vi "UpDownBinaryCounter12bitBreadmore.vi"() -> ()   [LabVIEW 2020]
panel:
  out "Decimal Decimal 2":dbl
  in  "Boolean 3":bool
  out "Boolean 2":bool
  out "Boolean":bool
  in  "Interval (sec)":dbl step=0.1
  out "7 3":bool
  out "7 2":bool
  out "7":bool
  out "6":bool
  out "5":bool
  out "4":bool
  out "3":bool
  out "2":bool
  out "1":bool
  out "0":bool
  # "12 bit Up Down Binary Counter\nAustin Breadmore"
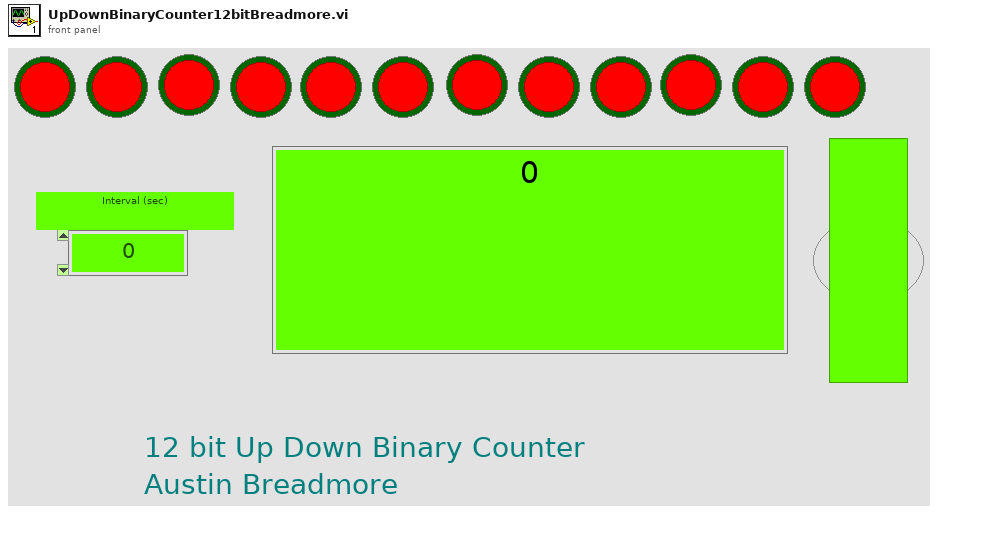
[diagram p1: front panel]
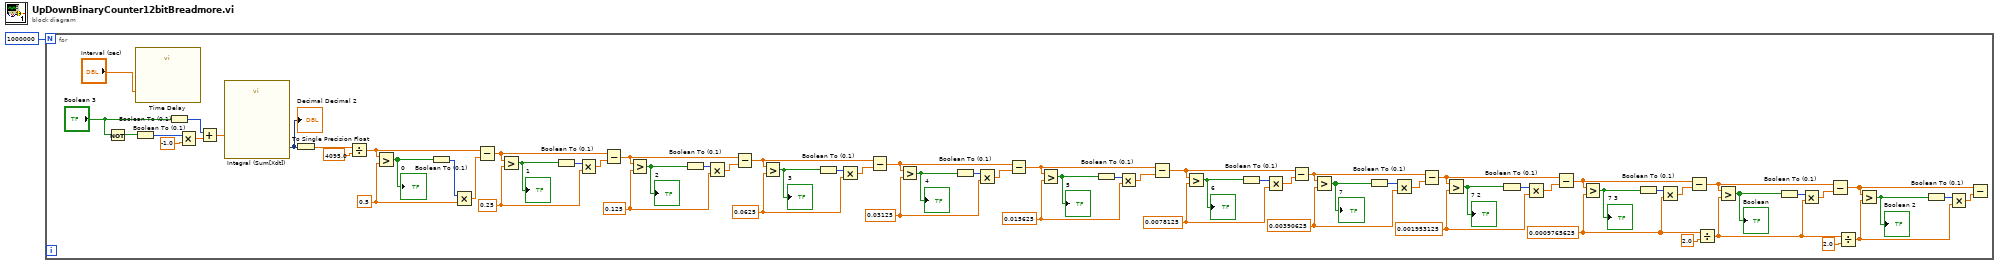
[diagram p0: block diagram]
diagram:
  n1 = for {
    N: 1000000 -> [_]
    w27 = 0.5 ("y")
    w20 = 0.0009765625 ("y")
    w34 = 0.001953125 ("y")
    w40 = 0.00390625 ("y")
    w44 = 0.0078125 ("y")
    w49 = 0.015625 ("y")
    w55 = 0.03125 ("y")
    w60 = 0.0625 ("y")
    w66 = 0.125 ("y")
    w71 = 0.25 ("y")
    n2 = Not(x="Boolean 3") -> (.not. x?=w8:bool)
    n3 = Boolean To (0,1)(Boolean=w8) -> (0, 1=w7:i16)
    n4 = call "Time Delay"("Delay Time (s)"="Interval (sec)") -> ()  [unwired: 10 in, 1 out]
    n5 = Boolean To (0,1)(Boolean="Boolean 3") -> (0, 1=w5:i16)
    n6 = Multiply(x=w7, y=-1.0) -> (x*y=w6:dbl)
    n7 = Add(x=w5, y=w6) -> (x+y=w4:dbl)
    n8 = call "Integral (Sum[Xdt])"("Signals"=w4) -> ("Result"=w2:dynamicdata)  [unwired: 5 in, 1 out]
    "Decimal Decimal 2" <- w2
    n9 = To Single Precision Float(number=w2) -> (single precision float=w3:sgl)
    n10 = Divide(x=w3, y=4095.0) -> (x/y=w26:dbl)
    n11 = Greater?(x=w26, y=w27) -> (0:w72:bool)
    "0" <- w72
    n12 = Boolean To (0,1)(Boolean=w72) -> (0, 1=w74:i16)
    n13 = Multiply(x=w74, y=w27) -> (x*y=w73:dbl)
    n14 = Subtract(x=w26, y=w73) -> (x-y=w69:dbl)
    n15 = Greater?(x=w69, y=w71) -> (0:w68:bool)
    "1" <- w68
    n16 = Boolean To (0,1)(Boolean=w68) -> (0, 1=w63:i16)
    n17 = Multiply(x=w63, y=w71) -> (x*y=w70:dbl)
    n18 = Subtract(x=w69, y=w70) -> (x-y=w64:dbl)
    n19 = Greater?(x=w64, y=w66) -> (0:w62:bool)
    "2" <- w62
    n20 = Boolean To (0,1)(Boolean=w62) -> (0, 1=w67:i16)
    n21 = Multiply(x=w67, y=w66) -> (x*y=w65:dbl)
    n22 = Subtract(x=w64, y=w65) -> (x-y=w58:dbl)
    n23 = Greater?(x=w58, y=w60) -> (0:w57:bool)
    "3" <- w57
    n24 = Boolean To (0,1)(Boolean=w57) -> (0, 1=w61:i16)
    n25 = Multiply(x=w61, y=w60) -> (x*y=w59:dbl)
    n26 = Subtract(x=w58, y=w59) -> (x-y=w53:dbl)
    n27 = Greater?(x=w53, y=w55) -> (0:w52:bool)
    "4" <- w52
    n28 = Boolean To (0,1)(Boolean=w52) -> (0, 1=w56:i16)
    n29 = Multiply(x=w56, y=w55) -> (x*y=w54:dbl)
    n30 = Subtract(x=w53, y=w54) -> (x-y=w48:dbl)
    n31 = Greater?(x=w48, y=w49) -> (0:w47:bool)
    "5" <- w47
    n32 = Boolean To (0,1)(Boolean=w47) -> (0, 1=w50:i16)
    n33 = Multiply(x=w50, y=w49) -> (x*y=w51:dbl)
    n34 = Subtract(x=w48, y=w51) -> (x-y=w42:dbl)
    n35 = Greater?(x=w42, y=w44) -> (0:w46:bool)
    "6" <- w46
    n36 = Boolean To (0,1)(Boolean=w46) -> (0, 1=w45:i16)
    n37 = Multiply(x=w45, y=w44) -> (x*y=w43:dbl)
    n38 = Subtract(x=w42, y=w43) -> (x-y=w39:dbl)
    n39 = Greater?(x=w39, y=w40) -> (0:w38:bool)
    "7" <- w38
    n40 = Boolean To (0,1)(Boolean=w38) -> (0, 1=w41:i16)
    n41 = Multiply(x=w41, y=w40) -> (x*y=w35:dbl)
    n42 = Subtract(x=w39, y=w35) -> (x-y=w33:dbl)
    n43 = Greater?(x=w33, y=w34) -> (0:w32:bool)
    "7 2" <- w32
    n44 = Boolean To (0,1)(Boolean=w32) -> (0, 1=w36:i16)
    n45 = Multiply(x=w36, y=w34) -> (x*y=w37:dbl)
    n46 = Subtract(x=w33, y=w37) -> (x-y=w30:dbl)
    n47 = Greater?(x=w30, y=w20) -> (0:w28:bool)
    "7 3" <- w28
    n48 = Boolean To (0,1)(Boolean=w28) -> (0, 1=w31:i16)
    n49 = Multiply(x=w31, y=w20) -> (x*y=w29:dbl)
    n50 = Subtract(x=w30, y=w29) -> (x-y=w19:dbl)
    n51 = Divide(x=w20, y=2.0) -> (x/y=w16:dbl)
    n52 = Greater?(x=w19, y=w16) -> (0:w18:bool)
    "Boolean" <- w18
    n53 = Boolean To (0,1)(Boolean=w18) -> (0, 1=w22:i16)
    n54 = Multiply(x=w22, y=w16) -> (x*y=w23:dbl)
    n55 = Subtract(x=w19, y=w23) -> (x-y=w13:dbl)
    n56 = Divide(x=w16, y=2.0) -> (x/y=w12:dbl)
    n57 = Greater?(x=w13, y=w12) -> (0:w11:bool)
    "Boolean 2" <- w11
    n58 = Boolean To (0,1)(Boolean=w11) -> (0, 1=w15:i16)
    n59 = Multiply(x=w15, y=w12) -> (x*y=w14:dbl)
    n60 = Subtract(x=w13, y=w14) -> ()  [unwired: 1 out]
  }
